vi "Maintenance v0.4.vi"(8 "Error In":errorcluster) -> (0 "Error out":errorcluster)   [LabVIEW 2021]
doc: "v0.4:\n- The cutting station CYL buttons are enabled only when both door SW are high"
uses:
  RT/Controls/DO 1.ctl
  Controls/Modbus Input.ctl
  GV/Maintenance GV.vi
panel:
  out "RS_Cutting_Rear":bool
  in  "Continuous?":bool
  in  "Main Tab":T1(tab)
  out "SW_Door_Front":bool
  out "Machine_ON":bool
  out "E_stop":bool
  out "SW_Pressure":bool
  out "SW_Start":bool
  out "SW_Reset":bool
  out "SW_Stop":bool
  out "SW_Door_Rear":bool
  in  "TL_Red":bool
  in  "TL_Orange":bool
  in  "TL_Green":bool
  in  "TL_Buzzer":bool
  in  "Index":bool
  in  "Start Index":bool
  in  "Index Timeout":i16
  in  "Index Position":i32
  in  "Index Software Torque Limit":u16
  in  "Index Hardware Torque Limit":u16
  out "Waveform Graph":i16[](graph)
  out "Index Time (ms)":u32
  out "RS_Index_Stopper _Rear":bool
  out "PES_Index_Pallet_Sensor":bool
  out "PES_Index_Output_Part Sensor":bool
  in  "Beckhoff Data":bool
  in  "Linear Feeder_2":bool
  in  "Linear Feeder_1":bool
  in  "Bowl  Feeder_ ON 2":bool
  out "ICS_BF_Pump_CNVR_Full_1":bool
  out "ICS_BF_Pump_CNVR_Full_2":bool
  out "ICS_BF_Pump_CNVR_Full_3":bool
  out "ICS_BF_Pump_CNVR_Full_4":bool
  in  "Bowl  Feeder_ ON 1":bool
  out "RS_Singling Rear":bool
  in  "Vaccuum OFF":bool
  in  "Vaccuum ON":bool
  in  "SOL_Singling":bool
  out "Vaccum Components Check":bool
  out "LS_Rotary_P&P":bool
  in  "SOL_Pick_Place_Rotary":bool
  out "PES_PC_Pump Presence_1":bool
  out "PES_PC_Pump Presence_2":bool
  out "PES_PC_Pump Presence_3":bool
  out "PES_PC_Pump Presence_4":bool
  out "RS_Pick_Place_Vertical":bool
  in  "SOL_Pick_Place_Vertical":bool
  out "PES_TF_Low_Level":bool
  out "RS_TF_Gating CYL_Rear":bool
  out "RS_Agitatator_1_Rear":bool
  in  "SOL_Tube_Feed_Agitator":bool
  in  "SOL_Tube_Feed_Gating_CYL":bool
  out "RS_Insertion_1_Rear":bool
  out "RS_Insertion_1_Front":bool
  out "RS_Insertion _2_Rear":bool
  out "RS_Insertion _2_Front":bool
  out "RS_Insertion _3_Rear":bool
  out "RS_Insertion _3_Front":bool
  out "RS_Insertion _4_Rear":bool
  out "RS_Insertion _4_Front":bool
  out "RS_Insertion_Clamp_Rear":bool
  in  "SOL_Insertion _CYL":bool
  in  "SOL_Insertion_Clamp_CYL":bool
  out "RS_Cutting_Forward_Rear":bool
  out "RS_Cutting_Rear3":bool
  out "RS_Cutting_Rear4":bool
  out "RS_Cutting_Rear1":bool
  out "RS_Cutting_Rear2":bool
  out "RS_Cutting_Clamp _Rear":bool
  in  "SOL_Cutting_CYL":bool
  in  "SOL_Cutting_Clamp_CYL":bool
  in  "SOL_Cutting_Forward_CYL":bool
  out "RS_Measurement__Rear":bool
  out "Distance Chart":T2(graph)
  out "IAS_MS_TubeLength_4":dbl caption="Sensor 4 (mm)" format="%#.3f"
  out "IAS_MS_TubeLength_3":dbl caption="Sensor 3 (mm)" format="%#.3f"
  out "IAS_MS_TubeLength_2":dbl caption="Sensor 2 (mm)" format="%#.3f"
  out "IAS_MS_TubeLength_1":dbl caption="Sensor 1 (mm)" format="%#.3f"
  out "RS_Measurement_ Front":bool
  in  "SOL_Measurement_CYL":bool
  out "RS_Rejection_1_Rear":bool
  out "RS_Rejection_2_Rear":bool
  out "RS_Rejection_3_Rear":bool
  out "RS_Rejection_4_Rear":bool
  in  "SOL_Rejection CYL_4":bool
  in  "SOL_Rejection CYL_3":bool
  in  "SOL_Rejection CYL_2":bool
  in  "SOL_Rejection CYL_1":bool
  in  "Velocity Mode":bool
  in  "Home":bool
  in  "Start":bool
  in  "Maintenance Position":i32
  in  "Maintenance Hardware Torque":u16
  in  "Homing Timeout":i16
  in  "Maintenance Software Torque":u16
  in  "Prehoming Position":i32
  in  "Prehoming Hardware Torque Limit":u16
  in  "Servo ON":bool
  in  "Start 2":bool
  in  "Stop":bool
  in  "Reset Fault":bool
  in  "Position Mode":bool
  in  "Maintenance Mode":bool
  in  "Prehoming Software Torque Limit":u16
  in  "Homing Position":i32
  in  "Homing Hardware Torque Limit":u16
  in  "Homing Software Torque Limit":u16
  in  "Close":bool
  # "Switches & Checks"
  # "Towerlight"
  # "Towerlight"
  # "Spare IO"
  # "Spare IO"
  # "Switches & Checks"
  # "Towerlight"
  # "Spare IO"
  # "Rotary Cylinder"
  # "Indexing"
  # "Stopper Cylinder"
  # "NOTE: This will perform a pre-defined indexing sequence while considering all safety inputs. In case of any error, no message will be shown on this screen; you will need to troubleshoot on Manual Mode."
  # "Other Inputs"
  # "Bowl Feeders"
  # "Bowl Feeder Track Full"
  # "Linear Feeder"
  # "Pump Conveyor Motor"
  # "Pump Presence Sensors"
  # "Gating Cylinder"
  # "Other IO"
  # "Agitator Cylinder"
  # "Tube Presence Sensors"
  # "Gating Cylinder"
  # "Other IO"
  # "Insertion Cylinders"
  # "Clamping Cylinder"
  # "Cutting Cylinder"
  # "Clamping Cylinder"
  # "Cutting Station"
  # "Switches & Checks"
  # "Distance Measurement"
  # "Rejection Cylinder 1"
  # "Rejection Cylinder 2"
  # "Rejection Cylinder 3"
  # "Rejection Cylinder 4"
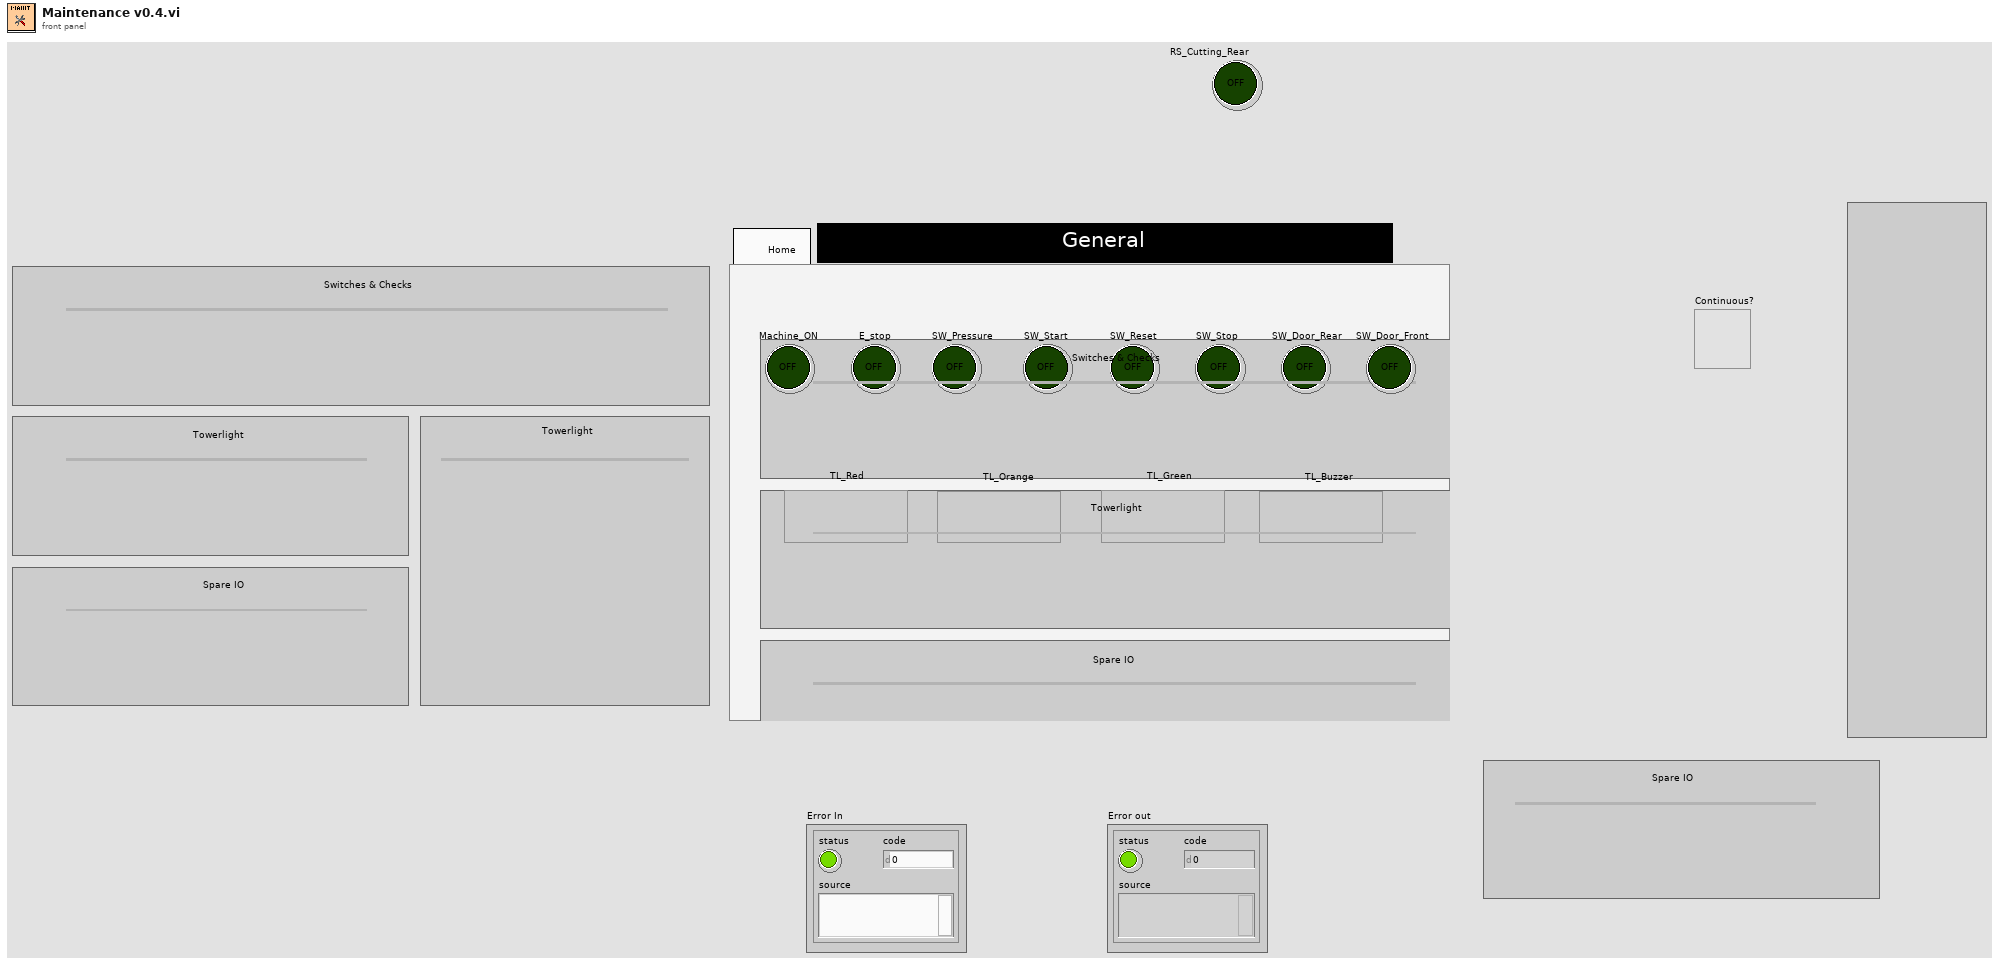
[diagram p1: front panel]
types:
  T1 = enum32{"General", "Indexing", "Bowl Feeders", "Pump Conveyor", "Tube Feeder", "Insertion Station", "Cutting Station", "Measurement Station", "Rejection Station", "Maintainence"}
  T2 = cluster{"IAS 1":dbl, "IAS 2":dbl, "IAS 3":dbl, "IAS 4":dbl}
  T3 = typedef "All Inputs.ctl" = cluster{"DI 1":T4, "DI 2":T5, "IAS 1":dbl, "IAS 2":dbl, "IAS 3":dbl, "IAS 4":dbl, "DO 1":T6}
  T4 = typedef "DI 1.ctl" = cluster{"Machine_ON":bool, "E_stop ":bool, "SW_Pressure":bool, "SW_Start ":bool, "SW_Reset":bool, "SW_Stop":bool, "SW_Door":bool, "Buffer 1":bool, "Buffer 2":bool, "RS_Index_Stopper _Rear":bool, "RS_Singling_Rear":bool, "IPS_Index_Pallet_Sensor":bool, "PES_Index_Output_Part Sensor":bool, "Buffer 3":bool, "SW_Cutting_Station_Door":bool, "PES_BF_Pump_CNVR_Full_1":bool, "PES_BF_Pump_CNVR_Full_2":bool, "PES_BF_Pump_CNVR_Full_3":bool, "PES_BF_Pump_CNVR_Full_4":bool, "PES_PC_Pump Presence_1":bool, "PES_PC_Pump Presence_2":bool, "PES_PC_Pump Presence_3":bool, "PES_PC_Pump Presence_4":bool, "RS_Pick_Place_Vertical":bool, "Buffer 5":bool, "PES_TF_Low_Level":bool, "RS_Cutting_Rear1":bool, "RS_Cutting_Rear2":bool, "RS_Cutting_Rear3":bool, "RS_Cutting_Rear4":bool, "RS_Cutting_Forward_Rear":bool, "Buffer 11":bool}
  T5 = typedef "DI 2.ctl" = cluster{"RS_Agitatator_1_Rear":bool, "Buffer 1 ":bool, "RS_TF_Gating CYL_Rear":bool, "RS_Insertion_1_Rear":bool, "RS_Insertion_1_Front":bool, "RS_Insertion _2_Rear":bool, "RS_Insertion _2_Front":bool, "RS_Insertion _3_Rear":bool, "RS_Insertion _3_Front":bool, "RS_Insertion _4_Rear":bool, "RS_Insertion _4_Front":bool, "RS_Insertion_Clamp_CYL":bool, "RS_Cutting_Rear":bool, "RS_Clamping_Rear":bool, "RS_Measurement_Front":bool, "RS_Measurement_Rear":bool, "Buffer 2":bool, "Buffer 3":bool, "Buffer 4":bool, "RS_Rejection_1_Rear":bool, "RS_Rejection_2_Rear":bool, "RS_Rejection_3_Rear":bool, "RS_Rejection_4_Rear":bool, "Buffer 5":bool, "Buffer 6":bool, "LS_Rotary_P&P":bool, "Vaccum Components check":bool, "Buffer 9":bool, "Buffer 10":bool, "Buffer 11":bool, "Buffer 12":bool, "Buffer 13":bool}
  T6 = typedef "DO 1.ctl" = cluster{"TL_Red":bool, "TL_Orange":bool, "TL_Green":bool, "TL_Buzzer":bool, "Vaccuum ON":bool, "Vaccuum OFF":bool, "Beckhoff Data":bool, "SOL_Singling":bool, "Bowl  Feeder_ ON 1":bool, "Buffer":bool, "SOL_Pick_Place_Vertical":bool, "SOL_Tube_Feed_Agitatator":bool, "SOL_Tube_Feed_Gating_CYL":bool, "SOL_Insertion _CYL":bool, "SOL_Insertion_Clamp_CYL":bool, "SOL_Cutting_CYL":bool, "SOL_Cutting_Clamp_CYL":bool, "SOL_Cutting_Foward_CYL":bool, "SOL_Measurement_CYL":bool, "SOL_Pick_Place_Rotary":bool, "SOL_Rejection CYL_1":bool, "SOL_Rejection CYL_2":bool, "SOL_Rejection CYL_3":bool, "SOL_Rejection CYL_4":bool, "Bowl  Feeder_ ON 2":bool, "Linear_Feeder 1":bool, "Linear_Feeder 2":bool, "Buffer 2":bool, "Buffer 3":bool, "Buffer 4":bool, "Buffer 5":bool, "Buffer 6":bool}
  T7 = enum8{"Enabled", "Disabled", "Disabled and Grayed Out"}
  T8 = typedef "Modbus Input.ctl" = cluster{"Maintenance Mode":bool, "Servo ON":bool, "Start":bool, "Stop":bool, "Reset Fault":bool, "Position Mode":bool, "Velocity Mode":bool, "Index":bool, "Start Index":bool, "Home":bool, "Start":bool, "Maintenance Position":i32, "Maintenance Hardware Torque":u16, "Maintenance Software Torque":u16, "Index Timeout":i16, "Index Position":i32, "Index Hardware Torque Limit":u16, "Index Software Torque Limit":u16, "Homing Timeout":i16, "Prehoming Position":i32, "Prehoming Hardware Torque Limit":u16, "Prehoming Software Torque Limit":u16, "Homing Position":i32, "Homing Hardware Torque Limit":u16, "Homing Software Torque Limit":u16}
  T9 = typedef "Index Details.ctl" = cluster{"Time (ms)":u32, "Waveform Graph":i16[]}
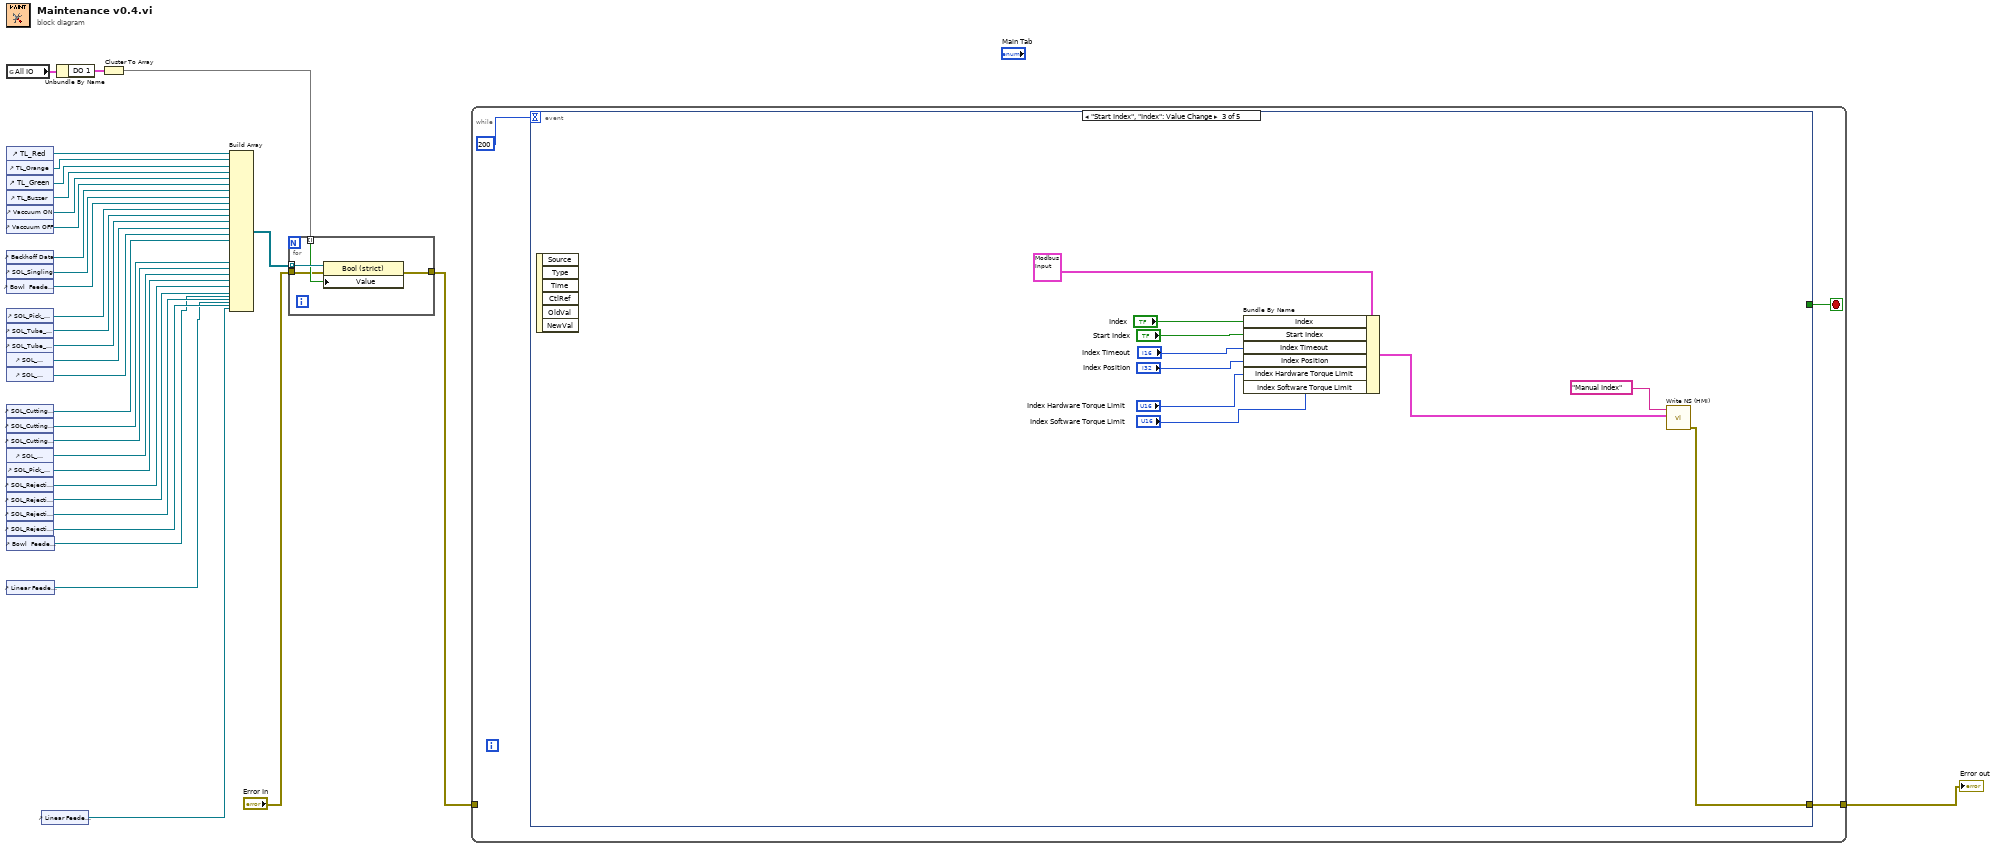
[diagram p0: block diagram]
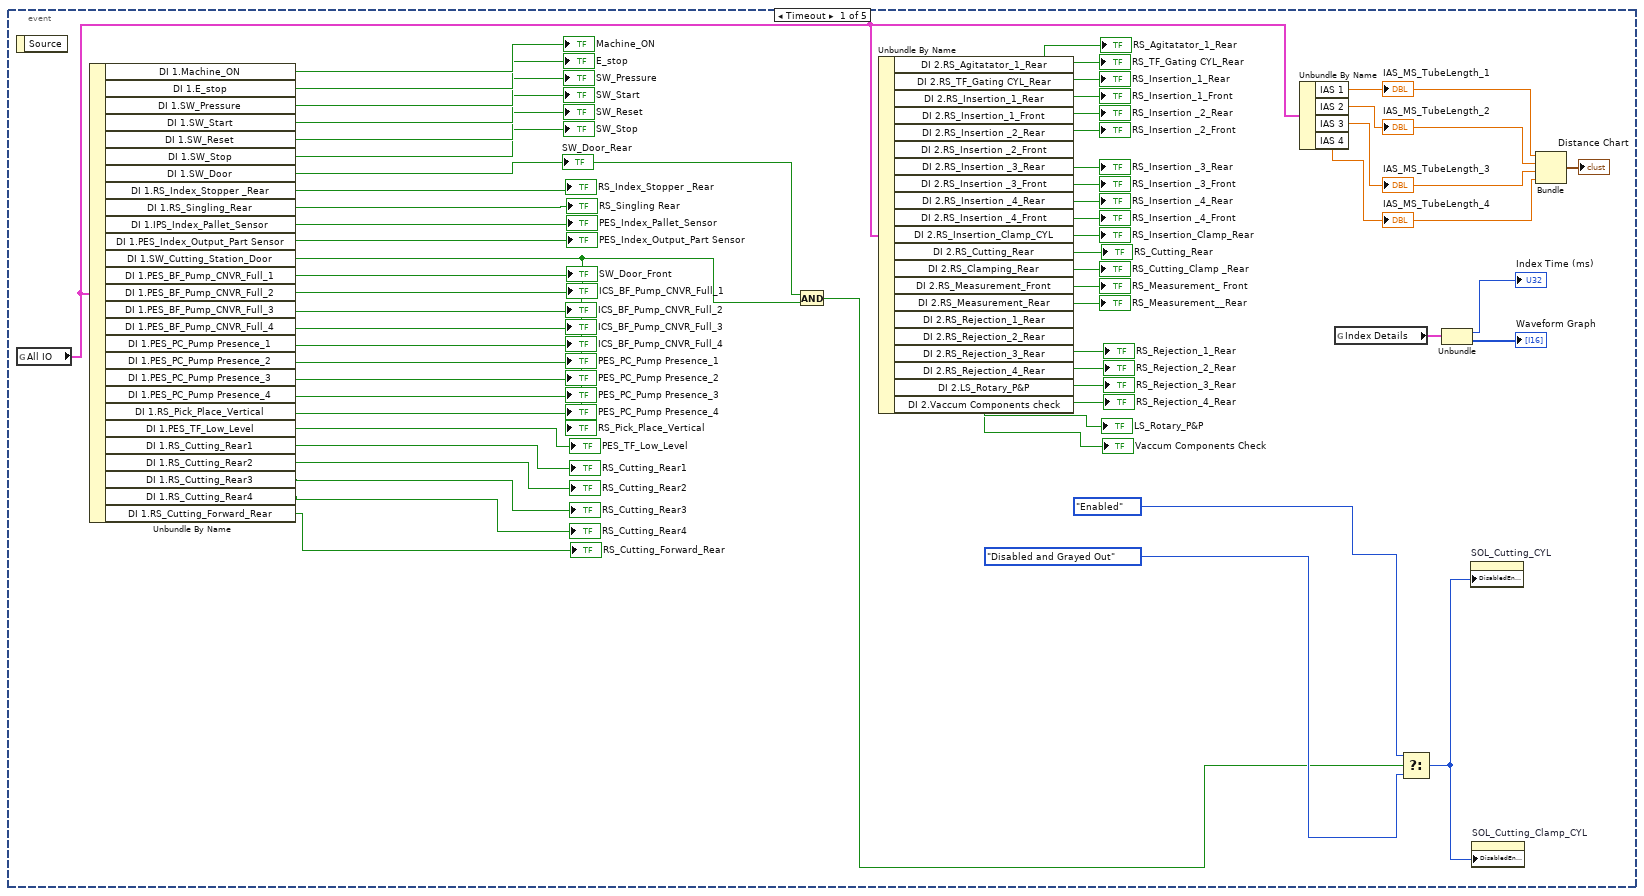
[diagram p2: hidden frame]
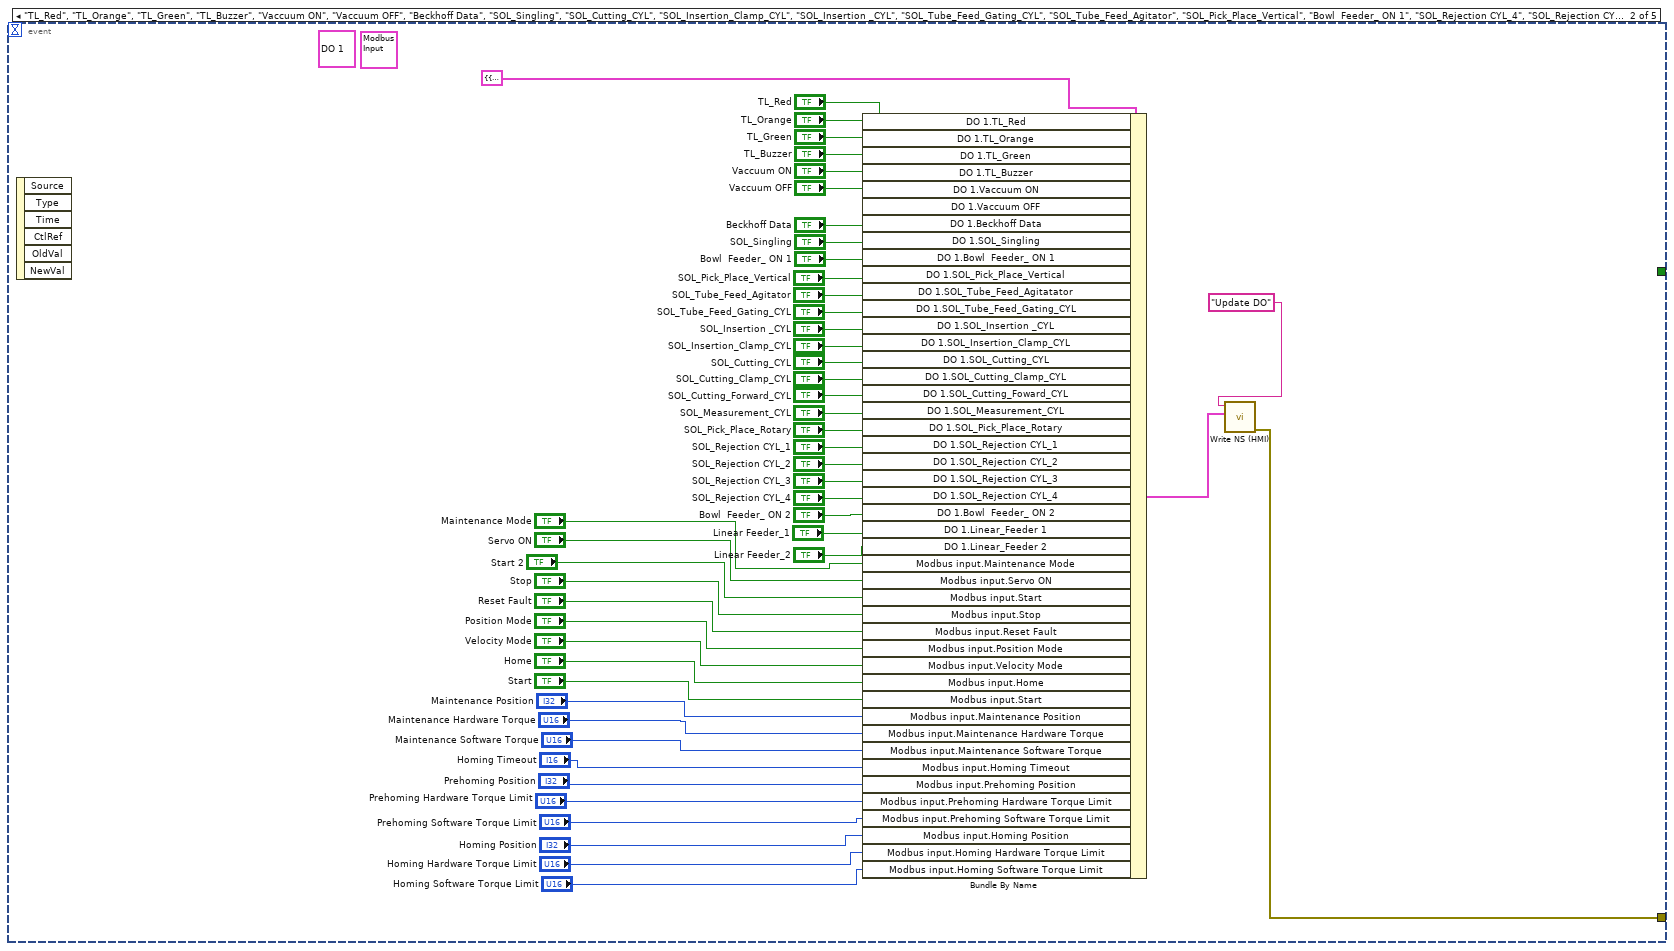
[diagram p3: hidden frame]
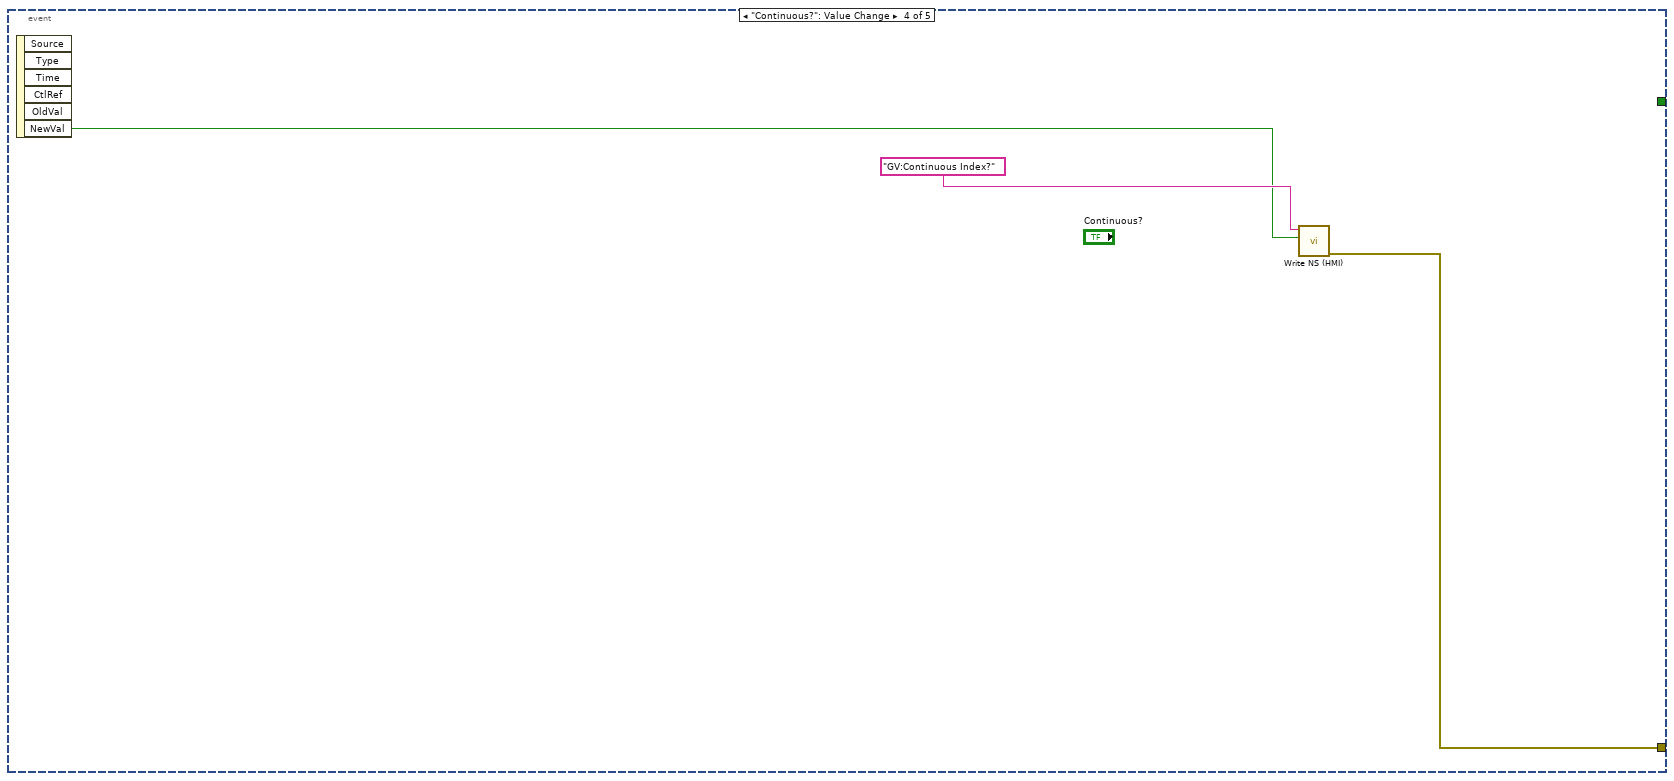
[diagram p4: hidden frame]
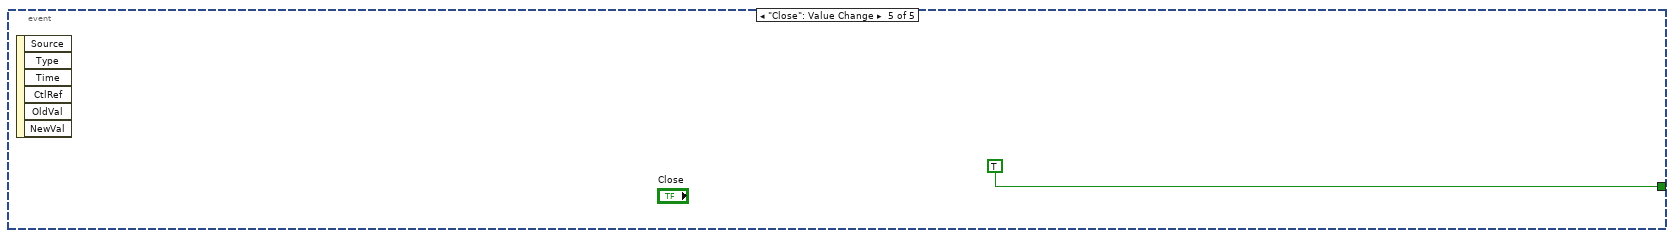
[diagram p5: hidden frame]
diagram:
  n1 = control-ref of="TL_Red"() -> (w33:refnum<vi>)
  n2 = control-ref of="TL_Orange"() -> (w32:refnum<vi>)
  n3 = control-ref of="TL_Green"() -> (w31:refnum<vi>)
  n4 = control-ref of="TL_Buzzer"() -> (w30:refnum<vi>)
  n5 = control-ref of="Vaccuum ON"() -> (w29:refnum<vi>)
  n6 = control-ref of="Vaccuum OFF"() -> (w28:refnum<vi>)
  n7 = control-ref of="Beckhoff Data"() -> (w27:refnum<vi>)
  n8 = control-ref of="SOL_Singling"() -> (w26:refnum<vi>)
  n9 = control-ref of="Bowl  Feeder_ ON 1"() -> (w25:refnum<vi>)
  n10 = control-ref of="SOL_Pick_Place_Vertical"() -> (w24:refnum<vi>)
  n11 = control-ref of="SOL_Tube_Feed_Agitator"() -> (w23:refnum<vi>)
  n12 = control-ref of="SOL_Tube_Feed_Gating_CYL"() -> (w22:refnum<vi>)
  n13 = control-ref of="SOL_Insertion _CYL"() -> (w21:refnum<vi>)
  n14 = control-ref of="SOL_Insertion_Clamp_CYL"() -> (w20:refnum<vi>)
  n15 = control-ref of="SOL_Cutting_CYL"() -> (w19:refnum<vi>)
  n16 = control-ref of="SOL_Cutting_Clamp_CYL"() -> (w18:refnum<vi>)
  n17 = control-ref of="SOL_Cutting_Forward_CYL"() -> (w17:refnum<vi>)
  n18 = control-ref of="SOL_Measurement_CYL"() -> (w16:refnum<vi>)
  n19 = control-ref of="SOL_Pick_Place_Rotary"() -> (w15:refnum<vi>)
  n20 = control-ref of="SOL_Rejection CYL_1"() -> (w14:refnum<vi>)
  n21 = control-ref of="SOL_Rejection CYL_2"() -> (w13:refnum<vi>)
  n22 = control-ref of="SOL_Rejection CYL_3"() -> (w12:refnum<vi>)
  n23 = control-ref of="SOL_Rejection CYL_4"() -> (w11:refnum<vi>)
  n24 = global read "Maintenance GV.vi" "All IO"() -> (w7:T3)
  n25 = control-ref of="Bowl  Feeder_ ON 2"() -> (w10:refnum<vi>)
  n26 = control-ref of="Linear Feeder_1"() -> (w9:refnum<vi>)
  n27 = control-ref of="Linear Feeder_2"() -> (w2:refnum<vi>)
  n28 = Unbundle By Name(w7) -> ("DO 1"=w6:T6)
  n29 = Cluster To Array(cluster=w6) -> (array=w5:bool[])
  n30 = Build Array(w33, w32, w31, w30, w29, w28, w27, w26, w25, w24, w23, w22, w21, w20, w19, w18, w17, w16, w15, w14, w13, w12, w11, w10, w9, w2) -> (w8:refnum<vi>[])
  n31 = for {
    tunnel: w8 -> [w37] mode=indexing
    tunnel: w5 -> [w36] mode=indexing
    tunnel: "Error In" -> [w35]
    tunnel: [w34] -> w3
    n32 = property class="Bool (strict)"(reference=w37, error in=w35, "Value"=w36) -> (error out=w34:errorcluster)  [unwired: 1 out]
  }
  n33 = while {
    tunnel: [w38] -> w1
    tunnel: w3 -> [_]
    stop <- w39 stop-if-true
    n34 = event shown="[2] \"Start Index\", \"Index\": Value Change" {
      selector: _ -> [_ _ _ _ _]
      dyn-events: _ -> [_ _ _ _ _]
      timeout: 200 -> [_ _ _ _ _]
      tunnel: [_ _ _ _ TRUE] -> w39
      tunnel: [_ w125 w159 w162 _] -> w38
      event Timeout {
        n35 = event-data() -> ()  [unwired: 1 in, 1 out]
        n36 = global read "Maintenance GV.vi" "All IO"() -> (w60:T3)
        n37 = Unbundle By Name(w60) -> ("DI 1.Machine_ON"=→"Machine_ON":bool, "DI 1.E_stop"=→"E_stop":bool, "DI 1.SW_Pressure"=→"SW_Pressure":bool, "DI 1.SW_Start"=→"SW_Start":bool, "DI 1.SW_Reset"=→"SW_Reset":bool, "DI 1.SW_Stop"=→"SW_Stop":bool, "DI 1.SW_Door"=w55:bool, "DI 1.RS_Index_Stopper _Rear"=→"RS_Index_Stopper _Rear":bool, "DI 1.RS_Singling_Rear"=→"RS_Singling Rear":bool, "DI 1.IPS_Index_Pallet_Sensor"=→"PES_Index_Pallet_Sensor":bool, "DI 1.PES_Index_Output_Part Sensor"=→"PES_Index_Output_Part Sensor":bool, "DI 1.SW_Cutting_Station_Door"=w56:bool, "DI 1.PES_BF_Pump_CNVR_Full_1"=→"ICS_BF_Pump_CNVR_Full_1":bool, "DI 1.PES_BF_Pump_CNVR_Full_2"=→"ICS_BF_Pump_CNVR_Full_2":bool, "DI 1.PES_BF_Pump_CNVR_Full_3"=→"ICS_BF_Pump_CNVR_Full_3":bool, "DI 1.PES_BF_Pump_CNVR_Full_4"=→"ICS_BF_Pump_CNVR_Full_4":bool, "DI 1.PES_PC_Pump Presence_1"=→"PES_PC_Pump Presence_1":bool, "DI 1.PES_PC_Pump Presence_2"=→"PES_PC_Pump Presence_2":bool, "DI 1.PES_PC_Pump Presence_3"=→"PES_PC_Pump Presence_3":bool, "DI 1.PES_PC_Pump Presence_4"=→"PES_PC_Pump Presence_4":bool, "DI 1.RS_Pick_Place_Vertical"=→"RS_Pick_Place_Vertical":bool, "DI 1.PES_TF_Low_Level"=→"PES_TF_Low_Level":bool, "DI 1.RS_Cutting_Rear1"=→"RS_Cutting_Rear1":bool, "DI 1.RS_Cutting_Rear2"=→"RS_Cutting_Rear2":bool, "DI 1.RS_Cutting_Rear3"=→"RS_Cutting_Rear3":bool, "DI 1.RS_Cutting_Rear4"=→"RS_Cutting_Rear4":bool, "DI 1.RS_Cutting_Forward_Rear"=→"RS_Cutting_Forward_Rear":bool)
        "SW_Door_Rear" <- w55
        "SW_Door_Front" <- w56
        n38 = And(x=w55, y=w56) -> (x .and. y?=w51:bool)
        n39 = Unbundle By Name(w60) -> ("DI 2.RS_Agitatator_1_Rear"=→"RS_Agitatator_1_Rear":bool, "DI 2.RS_TF_Gating CYL_Rear"=→"RS_TF_Gating CYL_Rear":bool, "DI 2.RS_Insertion_1_Rear"=→"RS_Insertion_1_Rear":bool, "DI 2.RS_Insertion_1_Front"=→"RS_Insertion_1_Front":bool, "DI 2.RS_Insertion _2_Rear"=→"RS_Insertion _2_Rear":bool, "DI 2.RS_Insertion _2_Front"=→"RS_Insertion _2_Front":bool, "DI 2.RS_Insertion _3_Rear"=→"RS_Insertion _3_Rear":bool, "DI 2.RS_Insertion _3_Front"=→"RS_Insertion _3_Front":bool, "DI 2.RS_Insertion _4_Rear"=→"RS_Insertion _4_Rear":bool, "DI 2.RS_Insertion _4_Front"=→"RS_Insertion _4_Front":bool, "DI 2.RS_Insertion_Clamp_CYL"=→"RS_Insertion_Clamp_Rear":bool, "DI 2.RS_Cutting_Rear"=→"RS_Cutting_Rear":bool, "DI 2.RS_Clamping_Rear"=→"RS_Cutting_Clamp _Rear":bool, "DI 2.RS_Measurement_Front"=→"RS_Measurement_ Front":bool, "DI 2.RS_Measurement_Rear"=→"RS_Measurement__Rear":bool, "DI 2.RS_Rejection_1_Rear"=→"RS_Rejection_1_Rear":bool, "DI 2.RS_Rejection_2_Rear"=→"RS_Rejection_2_Rear":bool, "DI 2.RS_Rejection_3_Rear"=→"RS_Rejection_3_Rear":bool, "DI 2.RS_Rejection_4_Rear"=→"RS_Rejection_4_Rear":bool, "DI 2.LS_Rotary_P&P"=→"LS_Rotary_P&P":bool, "DI 2.Vaccum Components check"=→"Vaccum Components Check":bool)
        n40 = Unbundle By Name(w60) -> ("IAS 1"=w94:dbl, "IAS 2"=w93:dbl, "IAS 3"=w92:dbl, "IAS 4"=w91:dbl)
        "IAS_MS_TubeLength_1" <- w94
        "IAS_MS_TubeLength_2" <- w93
        "IAS_MS_TubeLength_3" <- w92
        "IAS_MS_TubeLength_4" <- w91
        n41 = global read "Maintenance GV.vi" "Index Details"() -> (w59:T9)
        n42 = Select(t=T7."Enabled" ("Disabled"), s=w51, f=T7."Disabled and Grayed Out" ("Disabled")) -> (s? t:f=w52:T7)
        n43 = Unbundle(w59) -> ("Time (ms)"=→"Index Time (ms)":u32, "Waveform Graph"=→"Waveform Graph":i16[])
        n44 = property on="SOL_Cutting_CYL" class="Bool (strict)"("DisabledEnum"=w52) -> ()  [unwired: 2 in, 2 out]
        n45 = property on="SOL_Cutting_Clamp_CYL" class="Bool (strict)"("DisabledEnum"=w52) -> ()  [unwired: 2 in, 2 out]
        n46 = Bundle("IAS 1"=w94, "IAS 2"=w93, "IAS 3"=w92, "IAS 4"=w91) -> (→"Distance Chart":T2)  [unwired: 1 in]
      }
      event "TL_Red", "TL_Orange", "TL_Green", "TL_Buzzer", "Vaccuum ON", "Vaccuum OFF", "Beckhoff Data", "SOL_Singling", "SOL_Cutting_CYL", "SOL_Insertion_Clamp_CYL", "SOL_Insertion _CYL", "SOL_Tube_Feed_Gating_CYL", "SOL_Tube_Feed_Agitator", "SOL_Pick_Place_Vertical", "Bowl  Feeder_ ON 1", "SOL_Rejection CYL_4", "SOL_Rejection CYL_3", "SOL_Rejection CYL_2", "SOL_Rejection CYL_1", "SOL_Pick_Place_Rotary", "SOL_Measurement_CYL", "SOL_Cutting_Forward_CYL", "SOL_Cutting_Clamp_CYL", "Linear Feeder_1", "Bowl  Feeder_ ON 2", "Maintenance Mode", "Servo ON", "Start 2", "Stop", "Reset Fault", "Position Mode", "Velocity Mode", "Home", "Start", "Linear Feeder_2": Value Change {
        (unwired) T8 {"Maintenance Mode"=FALSE, "Servo ON"=FALSE, "Start"=FALSE, "Stop"=FALSE, "Reset Fault"=FALSE, "Position Mode"=FALSE, "Velocity Mode"=FALSE, "Index"=FALSE, "Start Index"=FALSE, "Home"=FALSE, "Start"=FALSE, "Maintenance Position"=0, "Maintenance Hardware Torque"=0, "Maintenance Software Torque"=0, "Index Timeout"=0, "Index Position"=0, "Index Hardware Torque Limit"=0, "Index Software Torque Limit"=0, "Homing Timeout"=0, "Prehoming Position"=0, "Prehoming Hardware Torque Limit"=0, "Prehoming Software Torque Limit"=0, "Homing Position"=0, "Homing Hardware Torque Limit"=0, "Homing Software Torque Limit"=0} ("Modbus input")
        (unwired) T6 {"TL_Red"=FALSE, "TL_Orange"=FALSE, "TL_Green"=FALSE, "TL_Buzzer"=FALSE, "Vaccuum ON"=FALSE, "Vaccuum OFF"=FALSE, "Beckhoff Data"=FALSE, "SOL_Singling"=FALSE, "Bowl  Feeder_ ON 1"=FALSE, "Buffer"=FALSE, "SOL_Pick_Place_Vertical"=FALSE, "SOL_Tube_Feed_Agitatator"=FALSE, "SOL_Tube_Feed_Gating_CYL"=FALSE, "SOL_Insertion _CYL"=FALSE, "SOL_Insertion_Clamp_CYL"=FALSE, "SOL_Cutting_CYL"=FALSE, "SOL_Cutting_Clamp_CYL"=FALSE, "SOL_Cutting_Foward_CYL"=FALSE, "SOL_Measurement_CYL"=FALSE, "SOL_Pick_Place_Rotary"=FALSE, "SOL_Rejection CYL_1"=FALSE, "SOL_Rejection CYL_2"=FALSE, "SOL_Rejection CYL_3"=FALSE, "SOL_Rejection CYL_4"=FALSE, "Bowl  Feeder_ ON 2"=FALSE, "Linear_Feeder 1"=FALSE, "Linear_Feeder 2"=FALSE, "Buffer 2"=FALSE, "Buffer 3"=FALSE, "Buffer 4"=FALSE, "Buffer 5"=FALSE, "Buffer 6"=FALSE} ("DO 1")
        n47 = event-data() -> ()  [unwired: 1 in, 6 out]
        n48 = Bundle By Name(cluster=cluster{"DO 1":T6, "Modbus input":T8} {"DO 1"={"TL_Red"=FALSE, "TL_Orange"=FALSE, "TL_Green"=FALSE, "TL_Buzzer"=FALSE, "Vaccuum ON"=FALSE, "Vaccuum OFF"=FALSE, "Beckhoff Data"=FALSE, "SOL_Singling"=FALSE, "Bowl  Feeder_ ON 1"=FALSE, "Buffer"=FALSE, "SOL_Pick_Place_Vertical"=FALSE, "SOL_Tube_Feed_Agitatator"=FALSE, "SOL_Tube_Feed_Gating_CYL"=FALSE, "SOL_Insertion _CYL"=FALSE, "SOL_Insertion_Clamp_CYL"=FALSE, "SOL_Cutting_CYL"=FALSE, "SOL_Cutting_Clamp_CYL"=FALSE, "SOL_Cutting_Foward_CYL"=FALSE, "SOL_Measurement_CYL"=FALSE, "SOL_Pick_Place_Rotary"=FALSE, "SOL_Rejection CYL_1"=FALSE, "SOL_Rejection CYL_2"=FALSE, "SOL_Rejection CYL_3"=FALSE, "SOL_Rejection CYL_4"=FALSE, "Bowl  Feeder_ ON 2"=FALSE, "Linear_Feeder 1"=FALSE, "Linear_Feeder 2"=FALSE, "Buffer 2"=FALSE, "Buffer 3"=FALSE, "Buffer 4"=FALSE, "Buffer 5"=FALSE, "Buffer 6"=FALSE}, "Modbus input"={"Maintenance Mode"=FALSE, "Servo ON"=FALSE, "Start"=FALSE, "Stop"=FALSE, "Reset Fault"=FALSE, "Position Mode"=FALSE, "Velocity Mode"=FALSE, "Index"=FALSE, "Start Index"=FALSE, "Home"=FALSE, "Start"=FALSE, "Maintenance Position"=0, "Maintenance Hardware Torque"=0, "Maintenance Software Torque"=0, "Index Timeout"=0, "Index Position"=0, "Index Hardware Torque Limit"=0, "Index Software Torque Limit"=0, "Homing Timeout"=0, "Prehoming Position"=0, "Prehoming Hardware Torque Limit"=0, "Prehoming Software Torque Limit"=0, "Homing Position"=0, "Homing Hardware Torque Limit"=0, "Homing Software Torque Limit"=0}}, "DO 1.TL_Red"="TL_Red", "DO 1.TL_Orange"="TL_Orange", "DO 1.TL_Green"="TL_Green", "DO 1.TL_Buzzer"="TL_Buzzer", "DO 1.Vaccuum ON"="Vaccuum ON", "DO 1.Vaccuum OFF"="Vaccuum OFF", "DO 1.Beckhoff Data"="Beckhoff Data", "DO 1.SOL_Singling"="SOL_Singling", "DO 1.Bowl  Feeder_ ON 1"="Bowl  Feeder_ ON 1", "DO 1.SOL_Pick_Place_Vertical"="SOL_Pick_Place_Vertical", "DO 1.SOL_Tube_Feed_Agitatator"="SOL_Tube_Feed_Agitator", "DO 1.SOL_Tube_Feed_Gating_CYL"="SOL_Tube_Feed_Gating_CYL", "DO 1.SOL_Insertion _CYL"="SOL_Insertion _CYL", "DO 1.SOL_Insertion_Clamp_CYL"="SOL_Insertion_Clamp_CYL", "DO 1.SOL_Cutting_CYL"="SOL_Cutting_CYL", "DO 1.SOL_Cutting_Clamp_CYL"="SOL_Cutting_Clamp_CYL", "DO 1.SOL_Cutting_Foward_CYL"="SOL_Cutting_Forward_CYL", "DO 1.SOL_Measurement_CYL"="SOL_Measurement_CYL", "DO 1.SOL_Pick_Place_Rotary"="SOL_Pick_Place_Rotary", "DO 1.SOL_Rejection CYL_1"="SOL_Rejection CYL_1", "DO 1.SOL_Rejection CYL_2"="SOL_Rejection CYL_2", "DO 1.SOL_Rejection CYL_3"="SOL_Rejection CYL_3", "DO 1.SOL_Rejection CYL_4"="SOL_Rejection CYL_4", "DO 1.Bowl  Feeder_ ON 2"="Bowl  Feeder_ ON 2", "DO 1.Linear_Feeder 1"="Linear Feeder_1", "DO 1.Linear_Feeder 2"="Linear Feeder_2", "Modbus input.Maintenance Mode"="Maintenance Mode", "Modbus input.Servo ON"="Servo ON", "Modbus input.Start"="Start 2", "Modbus input.Stop"="Stop", "Modbus input.Reset Fault"="Reset Fault", "Modbus input.Position Mode"="Position Mode", "Modbus input.Velocity Mode"="Velocity Mode", "Modbus input.Home"="Home", "Modbus input.Start"="Start", "Modbus input.Maintenance Position"="Maintenance Position", "Modbus input.Maintenance Hardware Torque"="Maintenance Hardware Torque", "Modbus input.Maintenance Software Torque"="Maintenance Software Torque", "Modbus input.Homing Timeout"="Homing Timeout", "Modbus input.Prehoming Position"="Prehoming Position", "Modbus input.Prehoming Hardware Torque Limit"="Prehoming Hardware Torque Limit", "Modbus input.Prehoming Software Torque Limit"="Prehoming Software Torque Limit", "Modbus input.Homing Position"="Homing Position", "Modbus input.Homing Hardware Torque Limit"="Homing Hardware Torque Limit", "Modbus input.Homing Software Torque Limit"="Homing Software Torque Limit") -> (w102:cluster{"DO 1":T6, "Modbus input":T8})
        n49 = call "Write NS (HMI).vi"("Message Data"=w102, "Message"="Update DO") -> ("error out"=w125:errorcluster)  [unwired: 9 in]
      }
      event "Start Index", "Index": Value Change {
        n50 = event-data() -> ()  [unwired: 1 in, 6 out]
        n51 = Bundle By Name(cluster=T8 {"Maintenance Mode"=FALSE, "Servo ON"=FALSE, "Start"=FALSE, "Stop"=FALSE, "Reset Fault"=FALSE, "Position Mode"=FALSE, "Velocity Mode"=FALSE, "Index"=FALSE, "Start Index"=FALSE, "Home"=FALSE, "Start"=FALSE, "Maintenance Position"=0, "Maintenance Hardware Torque"=0, "Maintenance Software Torque"=0, "Index Timeout"=0, "Index Position"=0, "Index Hardware Torque Limit"=0, "Index Software Torque Limit"=0, "Homing Timeout"=0, "Prehoming Position"=0, "Prehoming Hardware Torque Limit"=0, "Prehoming Software Torque Limit"=0, "Homing Position"=0, "Homing Hardware Torque Limit"=0, "Homing Software Torque Limit"=0} ("Modbus input"), "Index"="Index", "Start Index"="Start Index", "Index Timeout"="Index Timeout", "Index Position"="Index Position", "Index Hardware Torque Limit"="Index Hardware Torque Limit", "Index Software Torque Limit"="Index Software Torque Limit") -> (w156:T8)
        n52 = call "Write NS (HMI).vi"("Message Data"=w156, "Message"="Manual Index") -> ("error out"=w159:errorcluster)  [unwired: 9 in]
      }
      event "Continuous?": Value Change {
        n53 = event-data() -> ("NewVal"=w161:bool)  [unwired: 1 in, 5 out]
        n54 = call "Write NS (HMI).vi"("Message Data"=w161, "Message"="GV:Continuous Index?") -> ("error out"=w162:errorcluster)  [unwired: 9 in]
      }
      event "Close": Value Change {
        n55 = event-data() -> ()  [unwired: 1 in, 6 out]
      }
    }
  }
  "Error out" <- w1
